vi "read key value.vi"(8 "error in (no error)":errorcluster, 9 "key":string, 10 "section":string, 11 "Configuration File in":refnum<class "Configuration File.lvclass">) -> (0 "error out":errorcluster, 2 "value":string, 3 "Configuration File out":refnum<class "Configuration File.lvclass">)   [LabVIEW 2018, in "Configuration File.lvclass"]
uses:
  Configuration File.lvclass
  Configuration File.lvclass/Configuration File.ctl
  <vilib>/Utility/config.llb/Read Key (String).vi
  <vilib>/Utility/config.llb/NI_LVConfig.lvlib
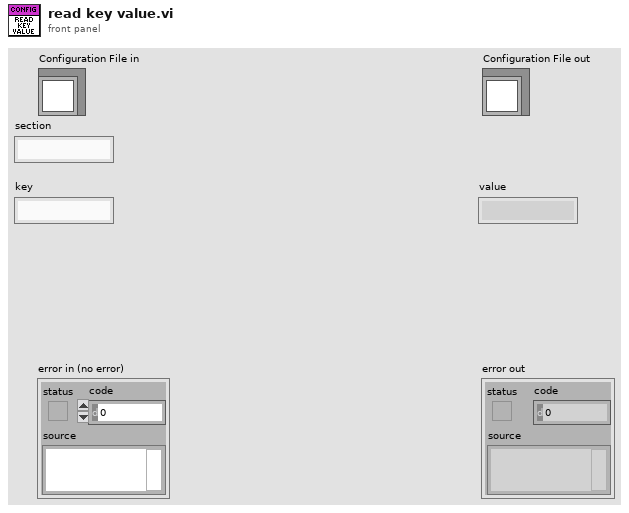
[diagram p1: front panel]
types:
  T1 = typedef "NI_LVConfig.lvlib/Config Data RefNum.ctl" = refnum<k1>
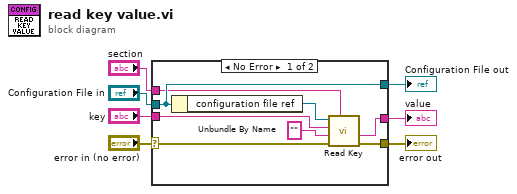
[diagram p0: block diagram]
diagram:
  n1 = case shown="No Error" "error in (no error)" {
    selector: "error in (no error)" -> [w15 w17]
    tunnel: [w14 w17] -> w6
    tunnel: [w13 w16] -> w4
    tunnel: "Configuration File in" -> [w13 w16]
    tunnel: [w10 _] -> w3
    tunnel: "section" -> [w9 _]
    tunnel: "key" -> [w8 _]
    frame No Error {
      n2 = Unbundle By Name(w13) -> ("configuration file ref"=w12:T1)
      n3 = call-poly <vilib>:"Read Key.vi"("section"=w9, "error in (no error)"=w15, "default value"="", "key"=w8, "refnum"=w12) -> ("error out"=w14:errorcluster, "value"=w10:string)  [unwired: 3 in, 2 out]
    }
    frame Error {
    }
  }
  "error out" <- w6
  "Configuration File out" <- w4
  "value" <- w3
